vi "XLP80_EA_ReadStatus_Batterie.vi"(8 "err in":errorcluster, 11 "Device information":string[](array[string])=["ASRL1::INSTR", "EL 3160-60 A", "000", "///", "1", "160", "60", "400", "10", "400"]) -> (0 "err out":errorcluster, 2 "Remote ON":bool, 3 "Device information IN":string[](array[string])=["ASRL1::INSTR", "EL 3160-60 A", "000", "///", "1", "160", "60", "400", "10", "400"])   [LabVIEW 2021]
uses:
  XLP80_EA_TDefsCluster_EA Feedback.ctl
  XLP80_EA_Globals.vi
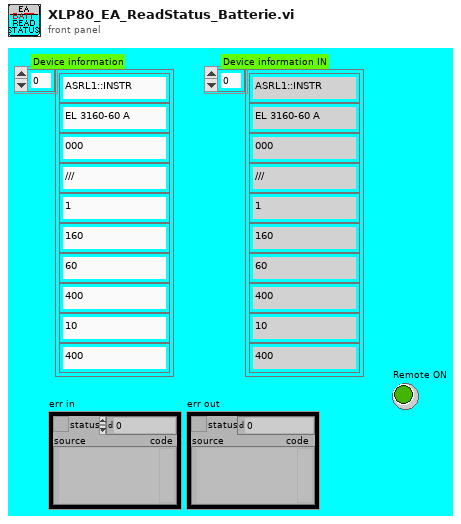
[diagram p1: front panel]
types:
  T1 = typedef "XLP80_EA_TDefsCluster_EA Feedback.ctl" = cluster{"EA on":bool, "Current":sgl, "Voltage":sgl, "Remote on":bool}
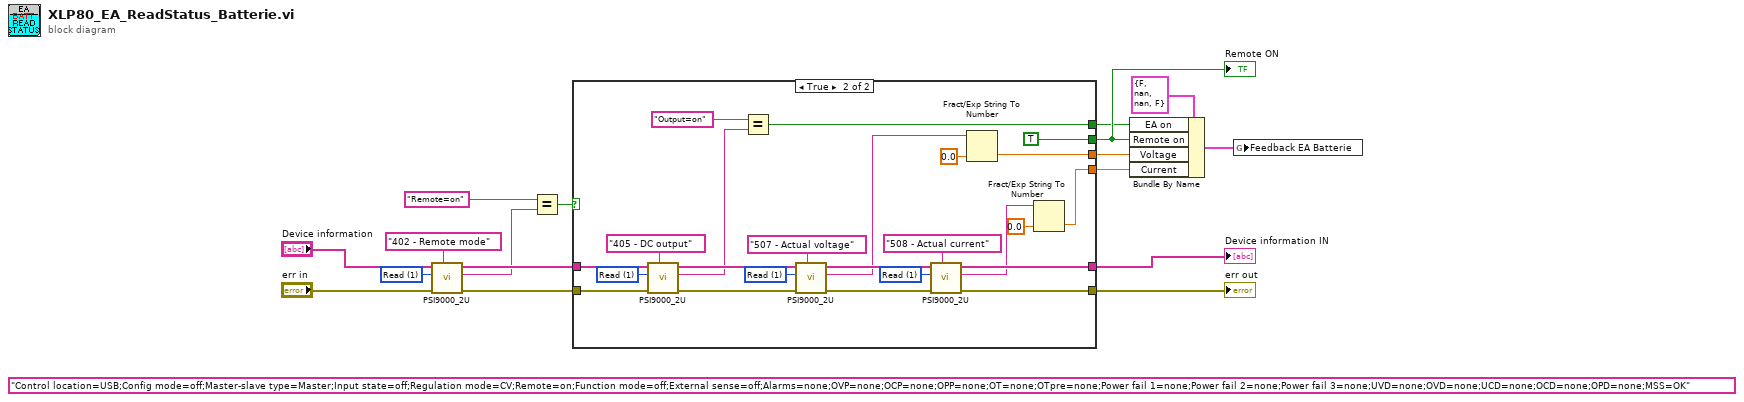
[diagram p0: block diagram]
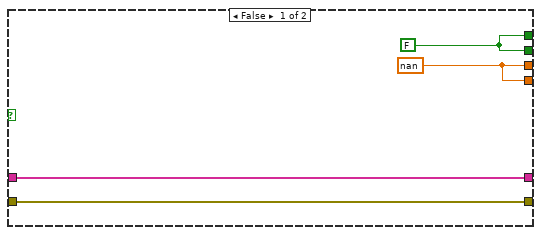
[diagram p2: hidden frame]
diagram:
  w11 = u8 1 items=["Write", "Read"] ("Access")
  (unwired) "Control location=USB;Config mode=off;Master-slave type=Master;Input state=off;Regulation mode=CV;Remote=on;Function mode=off;External sense=off;Alarms=none;OVP=none;OCP=none;OPP=none;OT=none;OTpre=none;Power fail 1=none;Power fail 2=none;Power fail 3=none;UVD=none;OVD=none;UCD=none;OCD=none;OPD=none;MSS=OK" ("Read data")
  n1 = call <instrlib>:"PSI9000_2U.vi"("Command list"="402 - Remote mode", "Error in"="err in", "Access"=w11, "Device information in"="Device information") -> ("Error out"=w9:errorcluster, "Read data"=w6:string, "Device information out"=w7:string[])  [unwired: 2 in, 1 out]
  n2 = Equal?(x="Remote=on", y=w6) -> (x = y?=w4:bool)
  n3 = case shown="True" w4 {
    tunnel: w7 -> [w20 w27]
    tunnel: w9 -> [w19 w29]
    tunnel: [w20 w40] -> w16
    tunnel: [w19 w39] -> w15
    tunnel: [w21 w35] -> w14
    tunnel: [w21 w32] -> w13
    tunnel: [w18 TRUE ("Remote on")] -> w3
    tunnel: [w18 w23] -> w2
    frame False {
      w21 = sgl nan
      w18 = FALSE ("Remote on")
    }
    frame True {
      w31 = u8 1 items=["Write", "Read"] ("Access")
      w43 = u8 1 items=["Write", "Read"] ("Access")
      w44 = u8 1 items=["Write", "Read"] ("Access")
      n4 = call <instrlib>:"PSI9000_2U.vi"("Command list"="405 - DC output", "Error in"=w29, "Access"=w31, "Device information in"=w27) -> ("Error out"=w28:errorcluster, "Read data"=w25:string, "Device information out"=w26:string[])  [unwired: 2 in, 1 out]
      n5 = Equal?(x="Output=on", y=w25) -> (x = y?=w23:bool)
      n6 = call <instrlib>:"PSI9000_2U.vi"("Command list"="507 - Actual voltage", "Error in"=w28, "Access"=w44, "Device information in"=w26) -> ("Error out"=w42:errorcluster, "Read data"=w37:string, "Device information out"=w41:string[])  [unwired: 2 in, 1 out]
      n7 = call <instrlib>:"PSI9000_2U.vi"("Command list"="508 - Actual current", "Error in"=w42, "Access"=w43, "Device information in"=w41) -> ("Error out"=w39:errorcluster, "Read data"=w33:string, "Device information out"=w40:string[])  [unwired: 2 in, 1 out]
      n8 = Fract/Exp String To Number(string=w37, default (0 dbl)=sgl 0.0 ("default (0 DBL)")) -> (number=w35:sgl)  [unwired: 2 in, 1 out]
      n9 = Fract/Exp String To Number(string=w33, default (0 dbl)=sgl 0.0 ("default (0 DBL)")) -> (number=w32:sgl)  [unwired: 2 in, 1 out]
    }
  }
  "err out" <- w15
  "Remote ON" <- w3
  "Device information IN" <- w16
  n10 = Bundle By Name(cluster=T1 {"EA on"=FALSE, "Current"=nan, "Voltage"=nan, "Remote on"=FALSE} ("Feedback EA Rekuperation"), "EA on"=w2, "Remote on"=w3, "Voltage"=w14, "Current"=w13) -> (w17:T1)
  n11 = global write "XLP80_EA_Globals.vi" "Feedback EA Batterie"(w17) -> ()
